vi "RC_Result Cluster User Event_UI.vi"(8 "error in (no error)":errorcluster, 10 "Result Cluster":T1, 11 "ZenGage v3.0 UI in":refnum<class "ZenGage v3.0 UI.lvclass">) -> (0 "error out":errorcluster, 3 "ZenGage v3.0 UI out":refnum<class "ZenGage v3.0 UI.lvclass">)   [LabVIEW 2019, in "ZenGage v3.0 UI.lvclass"]
uses:
  ZenGage v3.0 UI.lvclass
  <vilib>/vision/Image Controls.llb/IMAQ Image.ctl
  Type Definitions/Inspection/Result Cluster.ctl
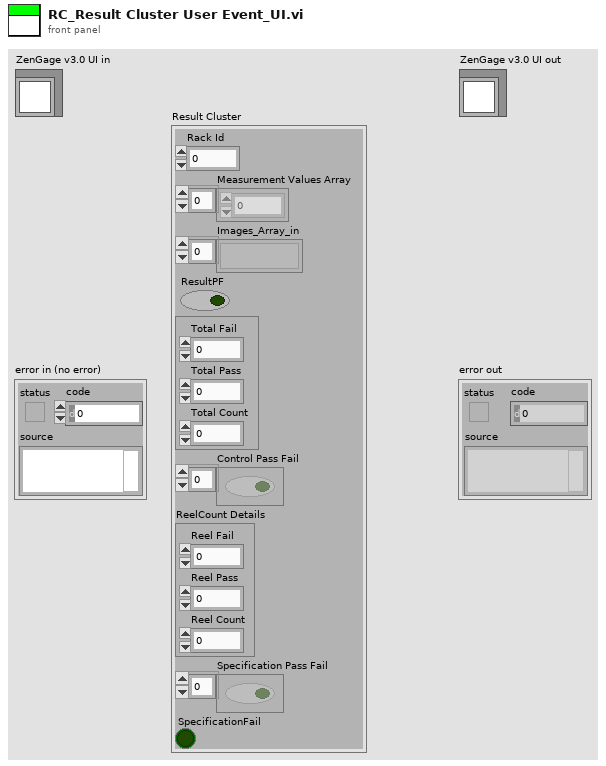
[diagram p1: front panel]
types:
  T1 = typedef "ZenGage v3.0 UI.lvclass/Result Cluster.ctl" = cluster{"Rack Id":u64, "Measurement Values Array ":dbl[], "Images_Array_in":T2[], "ResultPF":bool, "Production count details":cluster{"Total Count":dbl, "Total Pass":dbl, "Total Fail":dbl}, "Control Pass Fail":bool[], "ReelCount Details":cluster{"Reel Count":dbl, "Reel Pass":dbl, "Reel Fail":dbl}, "Specification Pass Fail":bool[], "SpecificationFail":bool}
  T2 = typedef "IMAQ Image.ctl" = refnum<image>
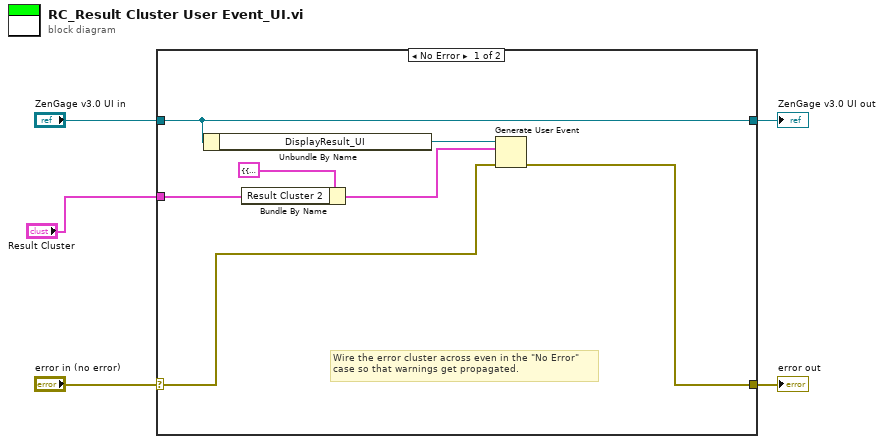
[diagram p0: block diagram]
diagram:
  n1 = case shown="No Error" "error in (no error)" {
    selector: "error in (no error)" -> [w10 w14]
    tunnel: [w9 w14] -> w4
    tunnel: [w12 w13] -> w2
    tunnel: "ZenGage v3.0 UI in" -> [w12 w13]
    tunnel: "Result Cluster" -> [w7 _]
    frame No Error {
      # "Wire the error cluster across even in the \"No Error\"\ncase so that warnings get propagated."
      n2 = Unbundle By Name(w12) -> ("DisplayResult_UI"=w11:refnum<user-event>)
      n3 = Bundle By Name(cluster=cluster{"Result Cluster 2":T1} {"Result Cluster 2"={"Rack Id"=0, "Measurement Values Array "=[], "Images_Array_in"=[], "ResultPF"=FALSE, "Production count details"={"Total Count"=0.0, "Total Pass"=0.0, "Total Fail"=0.0}, "Control Pass Fail"=[], "ReelCount Details"={"Reel Count"=0.0, "Reel Pass"=0.0, "Reel Fail"=0.0}, "Specification Pass Fail"=[], "SpecificationFail"=FALSE}} ("event data"), "Result Cluster 2"=w7) -> (w6:cluster{"Result Cluster 2":T1})
      n4 = Generate User Event(user event=w11, event data cluster=w6, error in=w10) -> (error out=w9:errorcluster)  [unwired: 1 in, 1 out]
    }
    frame Error {
    }
  }
  "error out" <- w4
  "ZenGage v3.0 UI out" <- w2
